vi "ForLoop.vi"() -> ()   [LabVIEW 2019]
panel:
  out "Iteration":i32
  in  "No of Iteration":i32
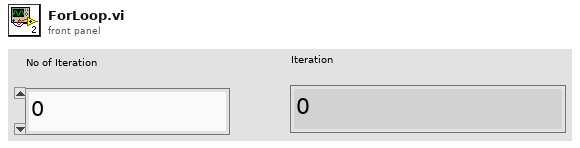
[diagram p1: front panel]
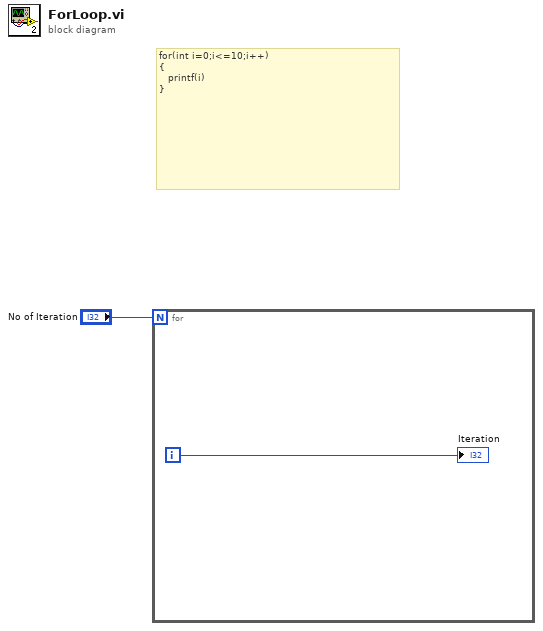
[diagram p0: block diagram]
diagram:
  # "for(int i=0;i<=10;i++)\n{\n   printf(i)\n}"
  n1 = for {
    N: "No of Iteration" -> [_]
    i -> [w2]
    "Iteration" <- w2
  }
